vi "board_1.vi"(0 "文件（使用对话框）":path, 8 "PWM1":dbl format="%0.2f") -> (18 "S1":dbl, 20 "S2":dbl, 21 "S3":dbl, 22 "S4":dbl, 23 "S5":dbl, 24 "S6":dbl, 25 "S7":dbl, 26 "S8":dbl, 27 "S9":dbl)   [LabVIEW 2017]
panel:
  out "sensor9":dbl[](array[numeric])
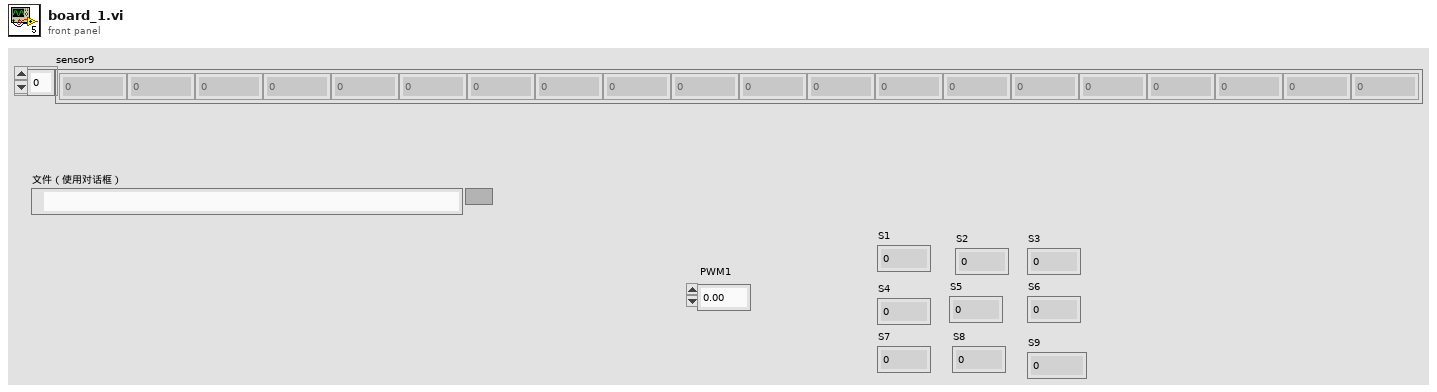
[diagram p1: front panel]
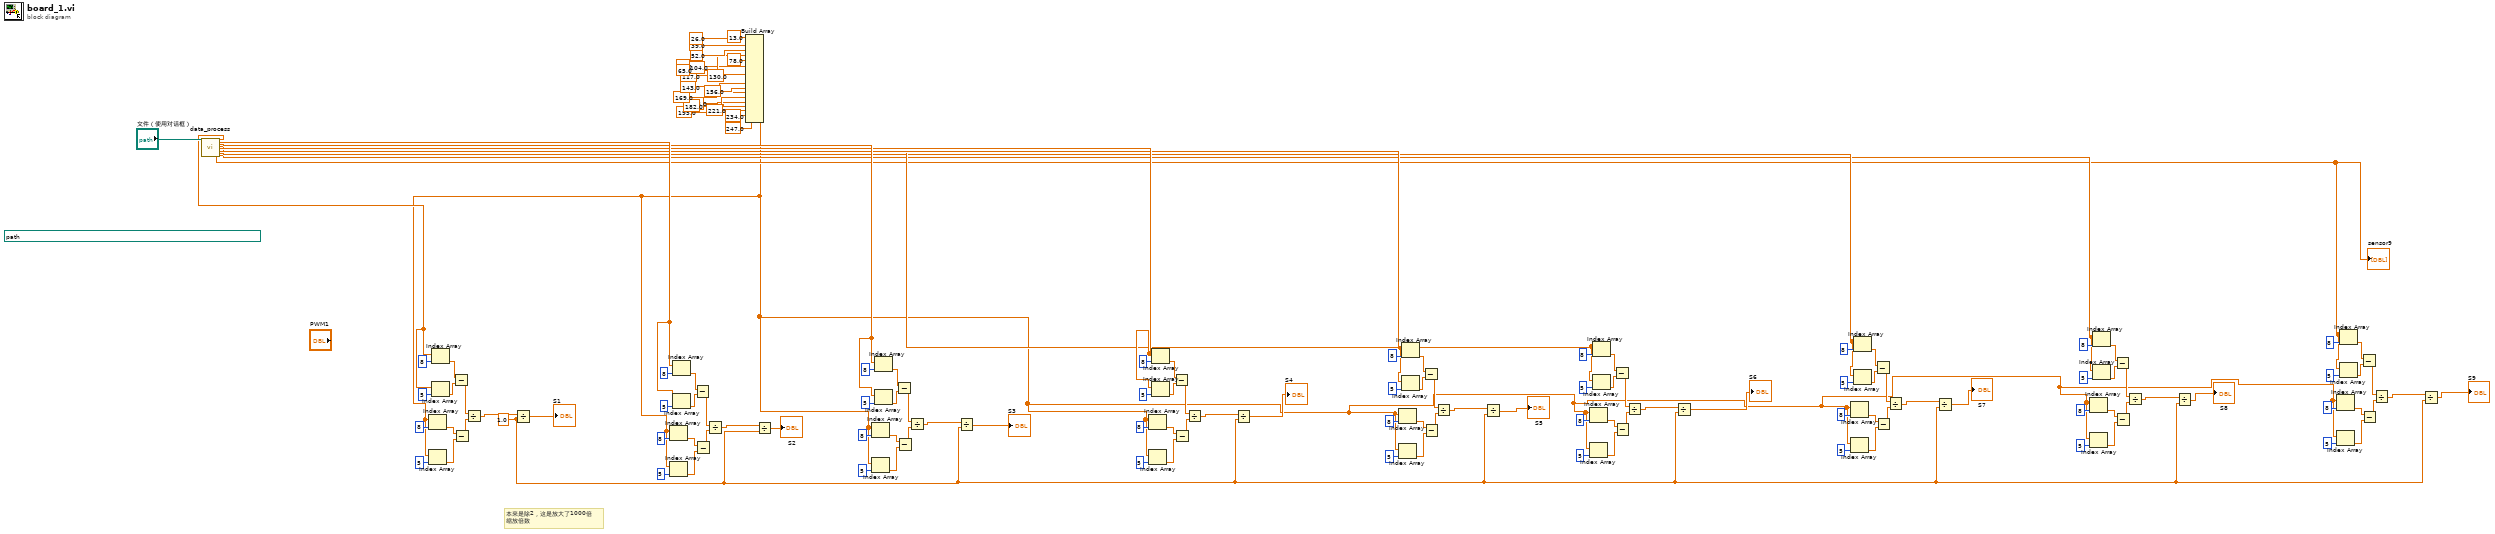
[diagram p0: block diagram]
diagram:
  w1 = 1.0 ("y")
  (unwired) path "D:/桌面文件/紫光传感器标定数据/程序/labview36/raw_data/S_rawdata_b1.txt" ("文件（使用对话框）")
  # "本来是除2，这是放大了1000倍\n缩放倍数"
  n1 = call "data_process.vi"("文件（使用对话框）"="文件（使用对话框）") -> ("SENSOR 9"=w4:dbl[], "SENSOR1"=w117:dbl[], "SENSOR 2"=w94:dbl[], "SENSOR 3"=w82:dbl[], "SENSOR 4"=w68:dbl[], "SENSOR 5"=w55:dbl[], "SENSOR 6"=w42:dbl[], "SENSOR 7"=w30:dbl[], "SENSOR 8"=w17:dbl[])  [unwired: 18 in]
  "sensor9" <- w4
  n2 = Index Array(array=w117, index=8 ("索引")) -> (element=w118:dbl)
  n3 = Index Array(array=w117, index=5 ("索引")) -> (element=w115:dbl)
  n4 = Subtract(x=w118, y=w115) -> (x-y=w114:dbl)
  n5 = Index Array(array=w94, index=8 ("索引")) -> (element=w97:dbl)
  n6 = Index Array(array=w94, index=5 ("索引")) -> (element=w99:dbl)
  n7 = Subtract(x=w97, y=w99) -> (x-y=w100:dbl)
  n8 = Build Array(13.0 ("元素"), 26.0 ("元素"), 39.0 ("元素"), 52.0 ("元素"), 65.0 ("元素"), 78.0 ("元素"), 91.0 ("元素"), 104.0 ("元素"), 117.0 ("元素"), 130.0 ("元素"), 143.0 ("元素"), 156.0 ("元素"), 169.0 ("元素"), 182.0 ("元素"), 195.0 ("元素"), 208.0 ("元素"), 221.0 ("元素"), 234.0 ("元素"), 247.0 ("元素")) -> (w3:dbl[])
  n9 = Index Array(array=w3, index=8 ("索引")) -> (element=w110:dbl)
  n10 = Index Array(array=w3, index=5 ("索引")) -> (element=w109:dbl)
  n11 = Subtract(x=w110, y=w109) -> (x-y=w113:dbl)
  n12 = Divide(x=w114, y=w113) -> (x/y=w108:dbl)
  n13 = Divide(x=w108, y=w1) -> (x/y=→"S1":dbl)
  n14 = Index Array(array=w3, index=8 ("索引")) -> (element=w104:dbl)
  n15 = Index Array(array=w3, index=5 ("索引")) -> (element=w105:dbl)
  n16 = Subtract(x=w104, y=w105) -> (x-y=w101:dbl)
  n17 = Divide(x=w100, y=w101) -> (x/y=w106:dbl)
  n18 = Divide(x=w106, y=w1) -> (x/y=→"S2":dbl)
  n19 = Index Array(array=w3, index=8 ("索引")) -> (element=w85:dbl)
  n20 = Index Array(array=w3, index=5 ("索引")) -> (element=w84:dbl)
  n21 = Index Array(array=w82, index=8 ("索引")) -> (element=w92:dbl)
  n22 = Index Array(array=w82, index=5 ("索引")) -> (element=w90:dbl)
  n23 = Subtract(x=w92, y=w90) -> (x-y=w89:dbl)
  n24 = Subtract(x=w85, y=w84) -> (x-y=w88:dbl)
  n25 = Divide(x=w89, y=w88) -> (x/y=w83:dbl)
  n26 = Divide(x=w83, y=w1) -> (x/y=→"S3":dbl)
  n27 = Index Array(array=w3, index=8 ("索引")) -> (element=w78:dbl)
  n28 = Index Array(array=w3, index=5 ("索引")) -> (element=w79:dbl)
  n29 = Index Array(array=w68, index=8 ("索引")) -> (element=w71:dbl)
  n30 = Index Array(array=w68, index=5 ("索引")) -> (element=w73:dbl)
  n31 = Subtract(x=w71, y=w73) -> (x-y=w74:dbl)
  n32 = Subtract(x=w78, y=w79) -> (x-y=w75:dbl)
  n33 = Divide(x=w74, y=w75) -> (x/y=w80:dbl)
  n34 = Divide(x=w80, y=w1) -> (x/y=→"S4":dbl)
  n35 = Index Array(array=w3, index=8 ("索引")) -> (element=w59:dbl)
  n36 = Index Array(array=w3, index=5 ("索引")) -> (element=w58:dbl)
  n37 = Index Array(array=w55, index=8 ("索引")) -> (element=w66:dbl)
  n38 = Index Array(array=w55, index=5 ("索引")) -> (element=w64:dbl)
  n39 = Subtract(x=w66, y=w64) -> (x-y=w63:dbl)
  n40 = Subtract(x=w59, y=w58) -> (x-y=w62:dbl)
  n41 = Divide(x=w63, y=w62) -> (x/y=w57:dbl)
  n42 = Divide(x=w57, y=w1) -> (x/y=→"S5":dbl)
  n43 = Index Array(array=w3, index=8 ("索引")) -> (element=w52:dbl)
  n44 = Index Array(array=w3, index=5 ("索引")) -> (element=w53:dbl)
  n45 = Index Array(array=w42, index=8 ("索引")) -> (element=w45:dbl)
  n46 = Index Array(array=w42, index=5 ("索引")) -> (element=w47:dbl)
  n47 = Subtract(x=w45, y=w47) -> (x-y=w48:dbl)
  n48 = Subtract(x=w52, y=w53) -> (x-y=w49:dbl)
  n49 = Divide(x=w48, y=w49) -> (x/y=w54:dbl)
  n50 = Divide(x=w54, y=w1) -> (x/y=→"S6":dbl)
  n51 = Index Array(array=w3, index=8 ("索引")) -> (element=w33:dbl)
  n52 = Index Array(array=w3, index=5 ("索引")) -> (element=w32:dbl)
  n53 = Index Array(array=w30, index=8 ("索引")) -> (element=w40:dbl)
  n54 = Index Array(array=w30, index=5 ("索引")) -> (element=w38:dbl)
  n55 = Subtract(x=w40, y=w38) -> (x-y=w37:dbl)
  n56 = Subtract(x=w33, y=w32) -> (x-y=w36:dbl)
  n57 = Divide(x=w37, y=w36) -> (x/y=w31:dbl)
  n58 = Divide(x=w31, y=w1) -> (x/y=→"S7":dbl)
  n59 = Index Array(array=w3, index=8 ("索引")) -> (element=w26:dbl)
  n60 = Index Array(array=w3, index=5 ("索引")) -> (element=w27:dbl)
  n61 = Index Array(array=w17, index=8 ("索引")) -> (element=w19:dbl)
  n62 = Index Array(array=w17, index=5 ("索引")) -> (element=w21:dbl)
  n63 = Subtract(x=w19, y=w21) -> (x-y=w22:dbl)
  n64 = Subtract(x=w26, y=w27) -> (x-y=w23:dbl)
  n65 = Divide(x=w22, y=w23) -> (x/y=w28:dbl)
  n66 = Divide(x=w28, y=w1) -> (x/y=→"S8":dbl)
  n67 = Index Array(array=w3, index=8 ("索引")) -> (element=w7:dbl)
  n68 = Index Array(array=w3, index=5 ("索引")) -> (element=w6:dbl)
  n69 = Index Array(array=w4, index=8 ("索引")) -> (element=w14:dbl)
  n70 = Index Array(array=w4, index=5 ("索引")) -> (element=w12:dbl)
  n71 = Subtract(x=w14, y=w12) -> (x-y=w11:dbl)
  n72 = Subtract(x=w7, y=w6) -> (x-y=w10:dbl)
  n73 = Divide(x=w11, y=w10) -> (x/y=w5:dbl)
  n74 = Divide(x=w5, y=w1) -> (x/y=→"S9":dbl)
